vi "daq_target.vi"() -> ()   [LabVIEW 2011]
uses:
  controls.llb/RTFIFO operate.ctl
  controls.llb/RTFIFO name.ctl
  controls.llb/data to RTFIFO.ctl
panel:
  out "x-y":u32
  out "output array":dbl[](array[numeric])
  out "size(s)":i32
  in  "stop":bool
  in  "data to RTFIFO":T1
  in  "variable":T2={"resource1"={"2503"="PXI1Slot3", "4070"="PXI1Slot2", "2530"=["PXI1Slot4", "PXI1Slot5", "PXI1Slot6", "PXI1Slot7", "PXI1Slot8", "PXI1Slot9", "PXI1Slot10"]}, "resource2"={"2503"="PXI1Slot12", "4070"="PXI1Slot11", "2530"=["PXI1Slot13", "PXI1Slot14", "PXI1Slot15"]}, "resource3"={"2530"="PXI1Slot17", "4070"="PXI1Slot16"}, "error"={"status"=FALSE, "code"=0, "source"=""}} {"error"."code" format="%.0x"}
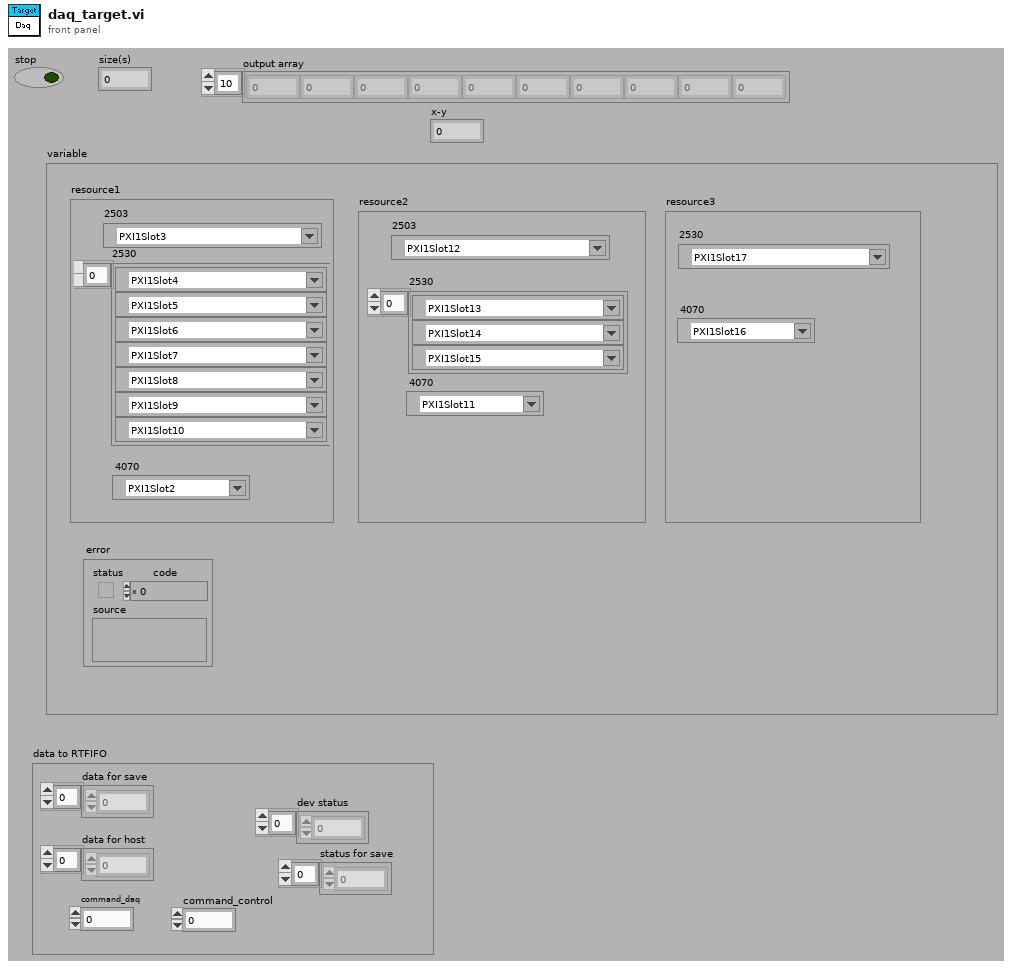
[diagram p1: front panel]
types:
  T1 = typedef "data to RTFIFO.ctl" = cluster{"data for save":dbl[], "data for host":dbl[], "command_daq":u16, "command_control":u16, "dev status":u16[], "status for save":u16[]}
  T2 = cluster{"resource1":cluster{"2503":refnum<k15>, "4070":refnum<k15>, "2530":refnum<k15>[]}, "resource2":cluster{"2503":refnum<k15>, "4070":refnum<k15>, "2530":refnum<k15>[]}, "resource3":cluster{"2530":refnum<k15>, "4070":refnum<k15>}, "error":errorcluster}
  T3 = typedef "RTFIFO name.ctl" = enum16{"command_daq", "command_control", "data for save", "data for host", "dev status", "status for save"}
  T4 = typedef "RTFIFO operate.ctl" = enum16{"Creat", "Write", "Read", "Delete"}
  T5 = typedef "data from RTFIFO.ctl" = cluster{"data for save":dbl[][], "data for host":dbl[][], "command_daq":u16, "command_control":u16, "dev status":u16[][], "status for save":u16[][]}
  T6 = cluster{"2503":refnum<k15>, "4070":refnum<k15>, "2530":refnum<k15>[]}
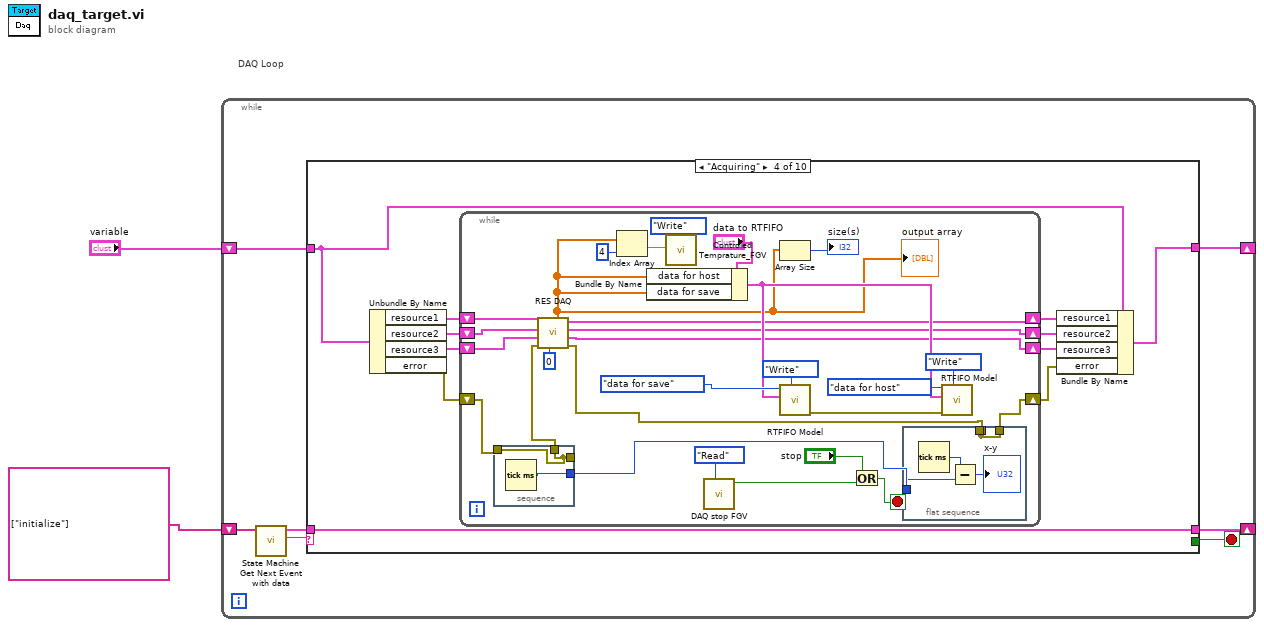
[diagram p0: block diagram]
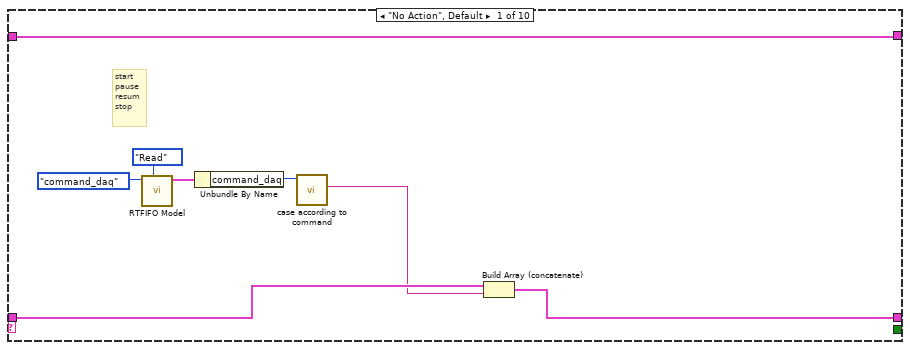
[diagram p2: hidden frame]
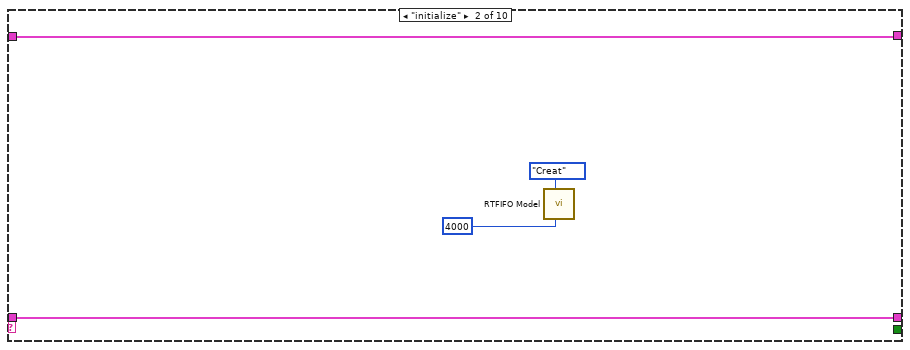
[diagram p3: hidden frame]
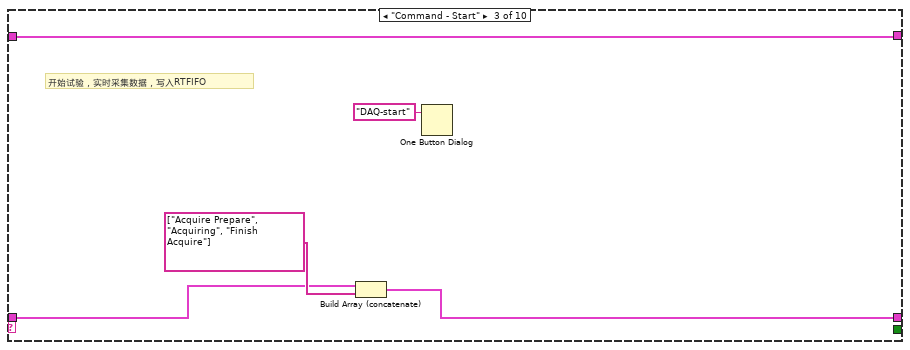
[diagram p4: hidden frame]
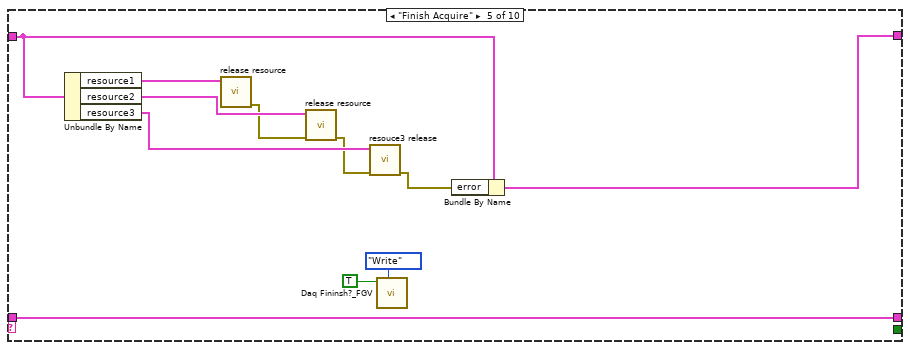
[diagram p5: hidden frame]
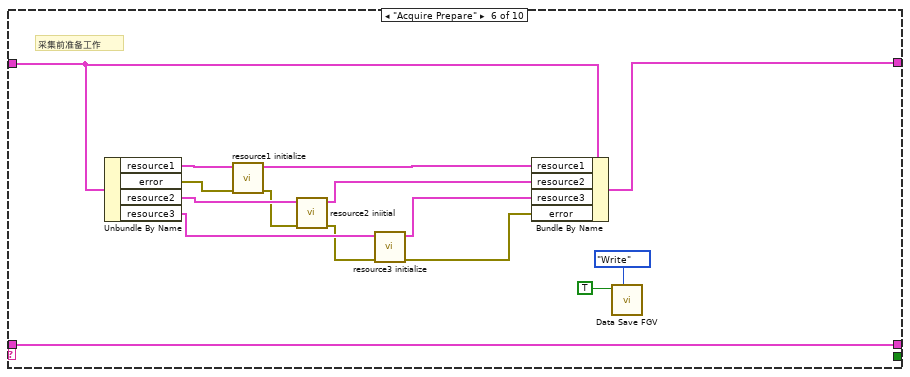
[diagram p6: hidden frame]
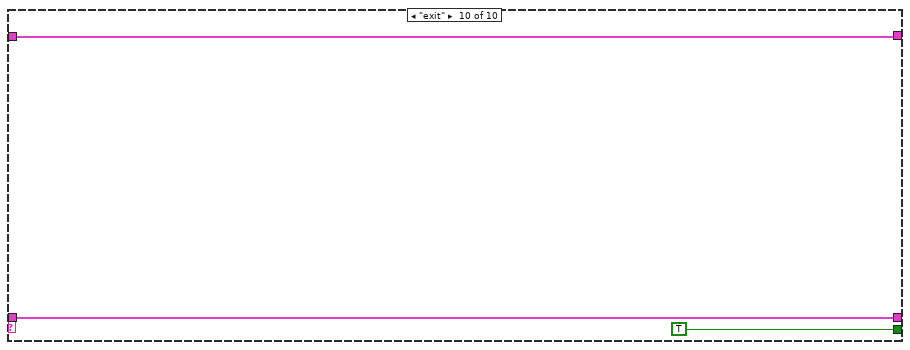
[diagram p10: hidden frame]
diagram:
  # "DAQ Loop"
  n1 = while {
    shift-right: [w6] -> _
    shift-left: string[] ["initialize"] -> [w9]
    shift-right: [w3] -> _
    shift-left: "variable" -> [w4]
    stop <- w5 stop-if-true
    n2 = call "State Machine Get Next Event with data.vi"("enent data queue in"=w9) -> ("next event"=w8:string, "event queue out"=w7:cluster{"event":string, "data":string}[])  [unwired: 5 in]
    n3 = case shown="\"Acquiring\"" w8 {
      tunnel: w7 -> [w17 w21 w24 w37 w81 w97 w99 w101 w103 w106]
      tunnel: [w16 w21 w23 w37 w81 w97 w99 w101 w103 w106] -> w6
      tunnel: [_ _ _ _ _ _ _ _ _ TRUE] -> w5
      tunnel: w4 -> [w10 w18 w22 w32 w73 w94 w98 w100 w102 w104]
      tunnel: [w10 w18 w22 w35 w72 w92 w98 w100 w102 w104] -> w3
      frame "No Action", Default {
        # "start\npause\nresum\nstop"
        n4 = call "RTFIFO Model.vi"("operate"=RTFIFO_operate."Read", "FIFO name"=RTFIFO_name."command_daq") -> ("data"=w13:T5)  [unwired: 8 in, 1 out]
        n5 = Unbundle By Name(w13) -> ("command_daq"=w12:u16)
        n6 = call "case according to command.vi"("command"=w12) -> ("case"=w11:string)  [unwired: 9 in, 1 out]
        n7 = Build Array (concatenate)(w17, w11) -> (w16:cluster{"event":string, "data":string}[])
      }
      frame "initialize" {
        n8 = call "RTFIFO Model.vi"("size"=4000, "operate"=RTFIFO_operate."Creat") -> ()  [unwired: 8 in, 2 out]
      }
      frame "Command - Start" {
        # "开始试验，实时采集数据，写入RTFIFO"
        n9 = Build Array (concatenate)(w24, string[] ["Acquire Prepare", "Acquiring", "Finish Acquire"] ("element")) -> (w23:cluster{"event":string, "data":string}[])
        n10 = One Button Dialog(message="DAQ-start") -> ()  [unwired: 1 in, 1 out]
      }
      frame "Acquiring" {
        n11 = Unbundle By Name(w32) -> ("resource1"=w36:T6, "resource2"=w34:T6, "resource3"=w33:cluster{"2530":refnum<k15>, "4070":refnum<k15>}, "error"=w31:errorcluster)
        n12 = while {
          shift-right: [w39] -> w30
          shift-left: w31 -> [w41]
          shift-right: [w50] -> w29
          shift-left: w36 -> [w47]
          shift-right: [w49] -> w28
          shift-left: w34 -> [w46]
          shift-right: [w48] -> w27
          shift-left: w33 -> [w45]
          stop <- w65 stop-if-true
          n13 = stacked-sequence {
            tunnel: [w67] -> w42
            tunnel: w41 -> [w66]
            tunnel: [w66] -> w40
            tunnel: [w66] -> _
            frame #0 {
              n14 = Tick Count (ms)() -> (millisecond timer value=w67:u32)
            }
          }
          n15 = call "RES DAQ.vi"("wendu #"=0, "error in"=w40, "resource3"=w45, "resouce2"=w46, "resource1"=w47) -> ("error out"=w38:errorcluster, "resource3 out"=w48:cluster{"2530":refnum<k15>, "4070":refnum<k15>}, "resouce2 out"=w49:T6, "resoure1 out"=w50:T6, "output array"=w44:dbl[])  [unwired: 1 in, 1 out]
          "output array" <- w44
          n16 = Index Array(array=w44, index=4) -> (element=w54:dbl)
          n17 = Bundle By Name(cluster="data to RTFIFO", "data for host"=w44, "data for save"=w44) -> (w55:T1)
          n18 = call "Controled Temprature_FGV.vi"("W/R"=enum16{"Write", "Read"}."Write", "Temprature in"=w54) -> ()  [unwired: 9 in, 1 out]
          n19 = call "DAQ stop FGV.vi"("W/R"=enum16{"Read", "Write"}."Read") -> ("stop ?"=w63:bool)  [unwired: 10 in]
          n20 = Array Size(array=w44) -> (size(s)=→"size(s)":i32)
          n21 = call "RTFIFO Model.vi"("operate"=RTFIFO_operate."Write", "data to RTFIFO"=w55, "FIFO name"=RTFIFO_name."data for save") -> ("error out"=w57:errorcluster)  [unwired: 7 in, 1 out]
          n22 = Or(x="stop", y=w63) -> (x .or. y?=w65:bool)
          n23 = flat-sequence {
            tunnel: w42 -> [w70]
            tunnel: w38 -> [w68]
            tunnel: [w68] -> _
            tunnel: [w68] -> w39
            frame #0 {
              n24 = Tick Count (ms)() -> (millisecond timer value=w71:u32)
              n25 = Subtract(x=w71, y=w70) -> (x-y=→"x-y":u32)
            }
          }
          n26 = call "RTFIFO Model.vi"("operate"=RTFIFO_operate."Write", "error in"=w57, "data to RTFIFO"=w55, "FIFO name"=RTFIFO_name."data for host") -> ()  [unwired: 6 in, 2 out]
        }
        n27 = Bundle By Name(cluster=w32, "resource1"=w29, "resource2"=w28, "resource3"=w27, "error"=w30) -> (w35:T2)
      }
      frame "Finish Acquire" {
        n28 = Unbundle By Name(w73) -> ("resource1"=w82:T6, "resource2"=w78:T6, "resource3"=w77:cluster{"2530":refnum<k15>, "4070":refnum<k15>})
        n29 = call "release resource.vi"("resource"=w82) -> ("error out"=w76:errorcluster)  [unwired: 10 in]
        n30 = call "release resource.vi"("error in"=w76, "resource"=w78) -> ("error out"=w75:errorcluster)  [unwired: 9 in]
        n31 = call "resouce3 release.vi"("error in"=w75, "resource3"=w77) -> ("error out"=w74:errorcluster)  [unwired: 9 in]
        n32 = call "Daq Fininsh?_FGV.vi"("W/R"=enum16{"Write", "Read"}."Write", "Daq Finish? in"=TRUE) -> ()  [unwired: 9 in, 1 out]
        n33 = Bundle By Name(cluster=w73, "error"=w74) -> (w72:T2)
      }
      frame "Acquire Prepare" {
        # "采集前准备工作"
        n34 = Unbundle By Name(w94) -> ("resource1"=w96:T6, "error"=w95:errorcluster, "resource2"=w91:T6, "resource3"=w88:cluster{"2530":refnum<k15>, "4070":refnum<k15>})
        n35 = call "resource1 initialize.vi"("error in"=w95, "resource1"=w96) -> ("error out"=w90:errorcluster, "resource1 out"=w93:T6)  [unwired: 8 in]
        n36 = call "resource2 iniitial.vi"("error in"=w90, "resource1"=w91) -> ("error out"=w87:errorcluster, "resource1 out"=w89:T6)  [unwired: 8 in]
        n37 = call "resource3 initialize.vi"("error in"=w87, "resource3"=w88) -> ("error out"=w85:errorcluster, "output cluster"=w86:cluster{"2530":refnum<k15>, "4070":refnum<k15>})  [unwired: 8 in]
        n38 = Bundle By Name(cluster=w94, "resource1"=w93, "resource2"=w89, "resource3"=w86, "error"=w85) -> (w92:T2)
        n39 = call "Data Save FGV .vi"("W/R"=enum16{"Read", "Write"}."Write", "Save?"=TRUE) -> ()  [unwired: 9 in, 1 out]
      }
      frame "Command - Pause" {
      }
      frame "Command - Resume" {
      }
      frame "Command - Stop" {
      }
      frame "exit" {
      }
    }
  }
